vi "Stereo - Global Variables.vi"() -> ()   [LabVIEW 2019]
doc: "Global Variable storing the Start Calibration Time and Start Live Image Time."
panel:
  out "Start Live Image Time":u32
  out "Start Calibration Time":u32
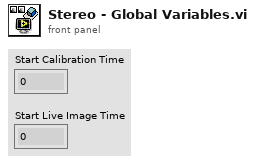
[diagram p1: front panel]
diagram:
